vi "lb-ft to N-m.vi"(11 "Torque (lb-ft)":sgl) -> (3 "Torque (N-m)":i16)   [LabVIEW 2020]
doc: "Converts torque from lb-ft to N-m. \n\nRounds single precision floating-point number to nearest integer and converts to 16-bit word integer."
panel:
  # "Torque Conversion"
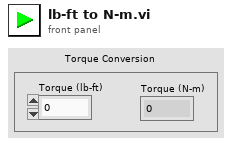
[diagram p1: front panel]
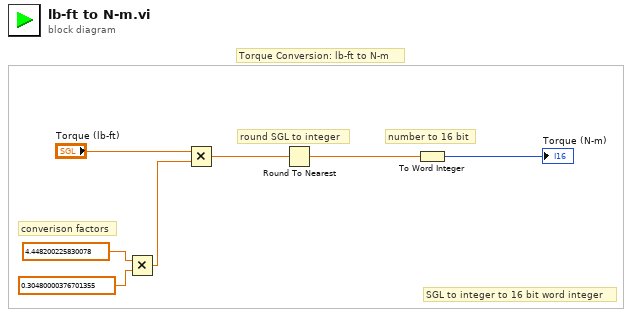
[diagram p0: block diagram]
diagram:
  # "Torque Conversion: lb-ft to N-m"
  # "SGL to integer to 16 bit word integer"
  # "number to 16 bit"
  # "round SGL to integer"
  # "converison factors"
  n1 = Multiply(x=sgl 4.4482, y=sgl 0.3048) -> (x*y=w4:sgl)
  n2 = Multiply(x="Torque (lb-ft)", y=w4) -> (x*y=w3:sgl)
  n3 = Round To Nearest(number=w3) -> (nearest integer value=w2:sgl)
  n4 = To Word Integer(number=w2) -> (16bit integer=→"Torque (N-m)":i16)
